vi "GlobalErrorCodes7.vi"(4 "Error Codes In":string[][](array[string]), 5 "Error Code In":string, 6 "Element #":i8, 7 "Function select":string) -> (0 "Error Codes Out":string[][](array[string]), 1 "Error Code Out":string[](array[string]), 2 "Error Name":string, 3 "Description":string)   [LabVIEW 2013]
uses:
  GlobalBoardIDs.vi
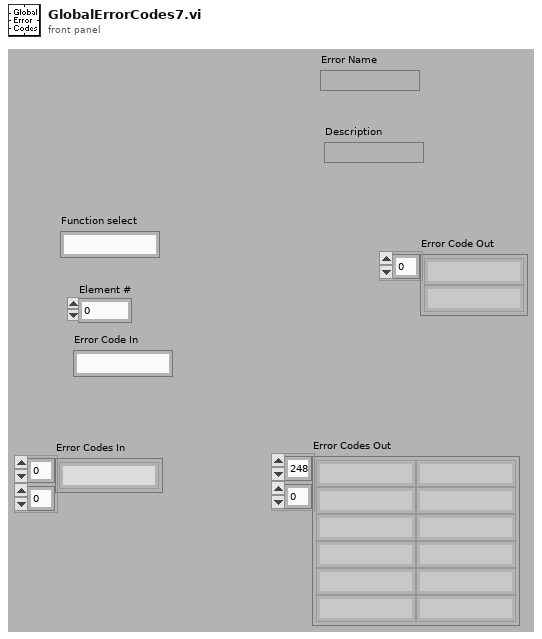
[diagram p1: front panel]
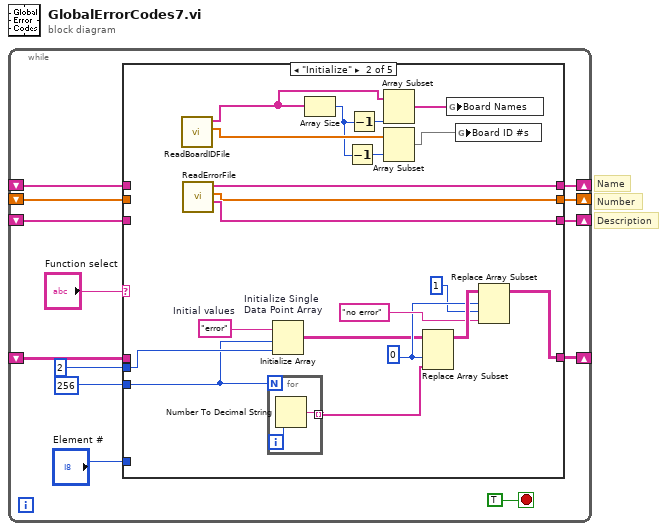
[diagram p0: block diagram]
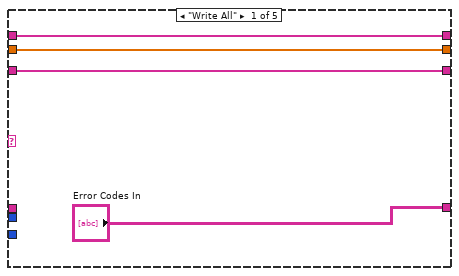
[diagram p2: hidden frame]
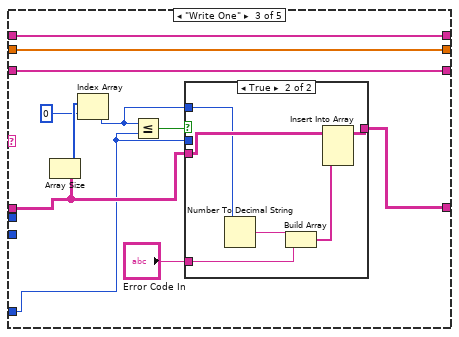
[diagram p3: hidden frame]
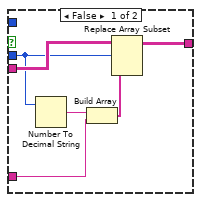
[diagram p4: hidden frame]
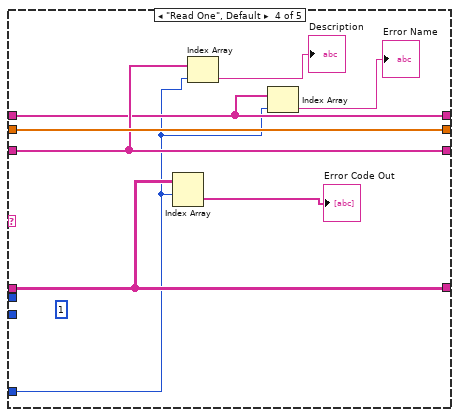
[diagram p5: hidden frame]
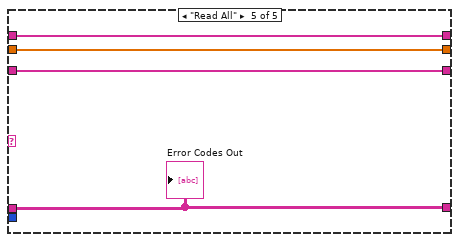
[diagram p6: hidden frame]
diagram:
  # "Description"
  # "Number"
  # "Name"
  n1 = while {
    shift-right: [w11] -> _
    shift-left: _ -> [w10]
    shift-right: [w6] -> _
    shift-left: _ -> [w3]
    shift-right: [w5] -> _
    shift-left: _ -> [w2]
    shift-right: [w4] -> _
    shift-left: _ -> [w1]
    stop <- TRUE stop-if-true
    n2 = case shown="\"Initialize\"" "Function select" {
      tunnel: 256 -> [_ w35 _ _ _]
      tunnel: ["Error Codes In" w28 w45 w70 w74] -> w11
      tunnel: w10 -> [_ _ w47 w70 w74]
      tunnel: "Element #" -> [_ _ w46 w64 _]
      tunnel: 2 -> [_ w36 _ _ _]
      tunnel: [w16 w26 w42 w65 w73] -> w6
      tunnel: [w15 w25 w41 w68 w72] -> w5
      tunnel: [w14 w27 w40 w67 w71] -> w4
      tunnel: w3 -> [w16 _ w42 w65 w73]
      tunnel: w2 -> [w15 _ w41 w68 w72]
      tunnel: w1 -> [w14 _ w40 w67 w71]
      frame "Write All" {
      }
      frame "Initialize" {
        w32 = 0
        w37 = "error"  # Initial values
        n3 = call "ReadBoardIDFile.vi"() -> ("Board Number"=w22:dbl[], "Board Name"=w23:string[])  [unwired: 9 in, 1 out]
        n4 = call "ReadErrorFile.vi"() -> ("Description"=w27:string[], "Error Number"=w25:dbl[], "Error Name"=w26:string[])  [unwired: 9 in]
        n5 = for {
          N: w35 -> [_]
          tunnel: [w38] -> w29 mode=indexing
          i -> [w39]
          n6 = Number To Decimal String(number=w39) -> (decimal integer string=w38:string)  [unwired: 1 in]
        }
        n7 = Initialize Array "Initialize Single\nData Point Array"(w37, w35, w36) -> (w30:string[][])
        n8 = Array Size(array=w23) -> (size(s)=w18:i32)
        n9 = Decrement(x=w18) -> (x-1=w20:i32)
        n10 = Decrement(x=w18) -> (x-1=w19:i32)
        n11 = Array Subset(array=w23, length=w19) -> (w24:string[])  [unwired: 1 in]
        n12 = Array Subset(array=w22, length=w20) -> (w21:dbl[])  [unwired: 1 in]
        n13 = Replace Array Subset(array=w30, new element=w29, index (col)=w32) -> (w34:string[][])  [unwired: 1 in]
        n14 = global write "GlobalBoardIDs.vi" "Board Names"(w24) -> ()
        n15 = global write "GlobalBoardIDs.vi" "Board ID #s"(w21) -> ()
        n16 = Replace Array Subset(array=w34, new element="no error", index (row)=w32, index (col)=1) -> (w28:string[][])
      }
      frame "Write One" {
        n17 = Array Size(array=w47) -> (size(s)=w49:i32[])
        n18 = Index Array(array=w49, index=0) -> (element=w43:i32)
        n19 = Less Or Equal?(x=w43, y=w46) -> (x <= y?=w50:bool)
        n20 = case shown="True" w50 {
          tunnel: w47 -> [w56 w62]
          tunnel: w46 -> [w54 _]
          tunnel: [w55 w61] -> w45
          tunnel: "Error Code In" -> [w52 w60]
          tunnel: w43 -> [_ w58]
          frame False {
            n21 = Number To Decimal String(number=w54) -> (decimal integer string=w53:string)  [unwired: 1 in]
            n22 = Build Array(w53, w52) -> (w51:string[])
            n23 = Replace Array Subset(array=w56, new element=w51, index (row)=w54) -> (w55:string[][])  [unwired: 1 in]
          }
          frame True {
            n24 = Number To Decimal String(number=w58) -> (decimal integer string=w57:string)  [unwired: 1 in]
            n25 = Build Array(w57, w60) -> (w59:string[])
            n26 = Insert Into Array(array=w62, new element=w59) -> (w61:string[][])  [unwired: 2 in]
          }
        }
      }
      frame "Read One", Default {
        (unwired) 1
        n27 = Index Array(array=w70, index (row)=w64) -> (element=→"Error Code Out":string[])  [unwired: 1 in]
        n28 = Index Array(array=w67, index=w64) -> (element=→"Description":string)
        n29 = Index Array(array=w65, index=w64) -> (element=→"Error Name":string)
      }
      frame "Read All" {
        "Error Codes Out" <- w74
      }
    }
  }
